vi "DPO_7K_Set_Acquisition_Mode.vi"(8 "Error In":errorcluster, 10 "Acquisition Mode":u16(ring) items=["Sample", "Peak Detect", "High resolution", "Average", "WFMDB", "Envelope"], 11 "VISA resource name in":refnum<visa-resource-name>) -> (0 "Error Out":errorcluster, 3 "VISA resource name out":refnum<visa-resource-name>)   [LabVIEW 2020]
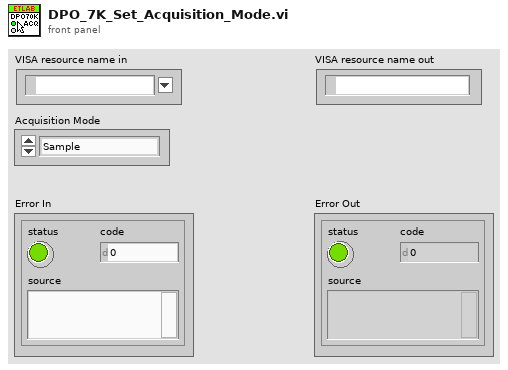
[diagram p1: front panel]
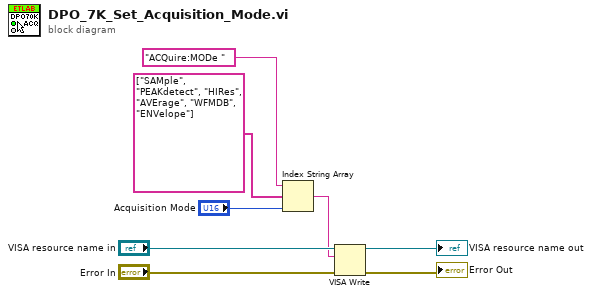
[diagram p0: block diagram]
diagram:
  n1 = Index String Array(1:"Acquisition Mode", 2:string[] ["SAMple", "PEAKdetect", "HIRes", "AVErage", "WFMDB", "ENVelope"], 3:"ACQuire:MODe ") -> (0:w1:string)
  n2 = VISA Write(VISA resource name="VISA resource name in", write buffer=w1, error in (no error)="Error In") -> (VISA resource name out=→"VISA resource name out":refnum<visa-resource-name>, error out=→"Error Out":errorcluster)  [unwired: 1 out]
